vi "1WIRE_Write_0_bit_multi.vi"(8 "error in":errorcluster, 11 "FPGA I/O":refnum<k21>="DS_WIRE") -> (0 "error out":errorcluster)   [LabVIEW 2014]
doc: "This VI is created by Vincent Claes for FPDA-1 more information on http://pwo.fpga.be\n\nvincent.claes@xios.be\nclaesvincent@gmail.com\n\nhttp://www.linkedin.com/in/vincentclaes"
uses:
  <vilib>/rvi/eio/common/nirviEmuTemplateMethod_errors.vi
  <vilib>/eio/EIOMethodNode/EIOMethodNode.xnode
  <vilib>/eio/EIONode/EIONode.xnode
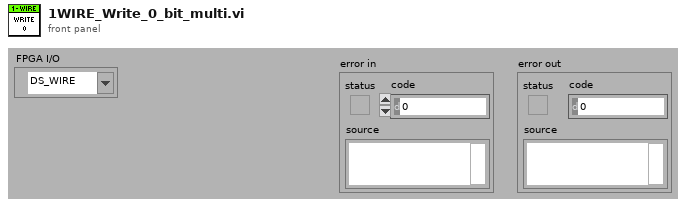
[diagram p1: front panel]
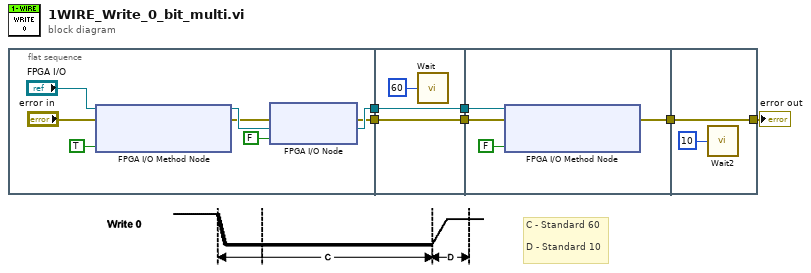
[diagram p0: block diagram]
diagram:
  # "C - Standard 60\n\nD - Standard 10"
  n1 = flat-sequence {
    tunnel: [w12] -> w6
    tunnel: [w9] -> w3
    tunnel: w6 -> [w16]
    tunnel: [w16] -> w5
    tunnel: [w15] -> w4
    tunnel: w3 -> [w15]
    tunnel: w5 -> [w20]
    tunnel: w4 -> [w19]
    tunnel: [w21] -> w2
    tunnel: [w22] -> w1
    tunnel: w2 -> [w22]
    frame #0 {
      n2 = xnode "FPGA I/O Method Node"("error in"="error in", "FPGA I/O In"="FPGA I/O", "Enable"=TRUE) -> ("error out"=w10:errorcluster, "FPGA I/O Out"=w13:refnum<k21>)
      n3 = xnode "FPGA I/O Node"("error in"=w10, "I/O Item"=FALSE ("FX2_IO1_J1_0"), "FPGA I/O In"=w13) -> ("error out"=w9:errorcluster, "FPGA I/O Out"=w12:refnum<k21>)
    }
    frame #1 {
      n4 = call "Wait"("Count(uSec)"=u32 60) -> ()  [unwired: 1 out]
    }
    frame #2 {
      n5 = xnode "FPGA I/O Method Node"("error in"=w19, "FPGA I/O In"=w20, "Enable"=FALSE) -> ("error out"=w21:errorcluster)  [unwired: 1 out]
    }
    frame #3 {
      n6 = call "Wait2"("Count(uSec)"=u32 10) -> ()  [unwired: 1 out]
    }
  }
  "error out" <- w1
